vi "Utility - Find Devices in Project.vi"(8 "error in (no error)":errorcluster caption="错误输入（无错误）", 11 "Device Tree Ref":refnum<vi> caption="设备树引用") -> (0 "error out":errorcluster caption="错误输出")   [LabVIEW 2015]
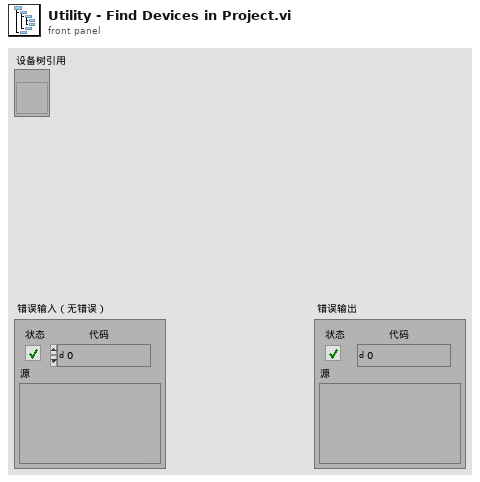
[diagram p1: front panel]
types:
  T1 = enum32{"None", "LabVIEW", "Mac OS", "Windows", "Default"}
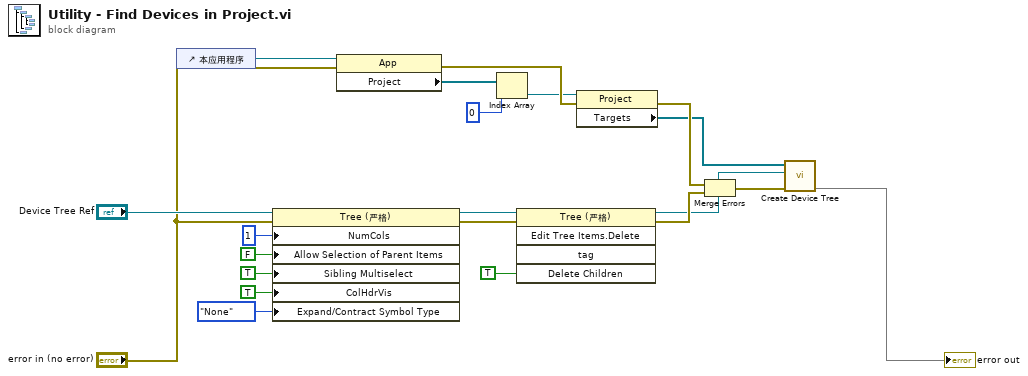
[diagram p0: block diagram]
diagram:
  n1 = control-ref of="本应用程序"() -> (w16:refnum<vi>)
  n2 = property class="Tree (严格)"(reference="Device Tree Ref", error in="error in (no error)", "NumCols"=u32 1 ("列数"), "Allow Selection of Parent Items"=FALSE ("允许选择父项"), "Sibling Multiselect"=TRUE ("同辈多选"), "ColHdrVis"=TRUE ("允许选择父项"), "Expand/Contract Symbol Type"=T1."None" ("缩进/移出符号:符号类型")) -> (reference out=w11:refnum<vi>, error out=w10:errorcluster)
  n3 = property class="App"(reference=w16, error in="error in (no error)") -> (error out=w19:errorcluster, "Project"=w20:refnum<vi>[])  [unwired: 1 out]
  n4 = Index Array(array=w20, index=0 ("索引")) -> (element=w18:refnum<vi>)
  n5 = invoke class="Tree (严格)" method="Edit Tree Items.Delete"(reference=w11, error in=w10, "Delete Children"=TRUE ("删除子项？")) -> (reference out=w1:refnum<vi>, error out=w6:errorcluster)  [unwired: 2 in, 3 out]
  n6 = property class="Project"(reference=w18, error in=w19) -> (error out=w3:errorcluster, "Targets"=w2:refnum<vi>[])  [unwired: 1 out]
  n7 = Merge Errors(w3, w6) -> (w4:errorcluster)
  n8 = call "Create Device Tree.vi"(8:w4, "Device Tree Items"=w1, "Device Tree Ref"=w2) -> (0:→"error out")  [unwired: 8 in]
